vi "FG LED.vi"(2 "FG Action":T1, 3 "LED in":bool) -> (1 "LED out":bool)   [LabVIEW 2009]
uses:
  cRIO/Functional Global Variables/Actions for FG's.ctl
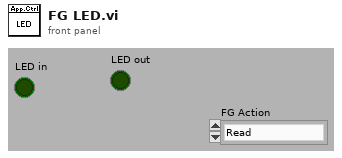
[diagram p1: front panel]
types:
  T1 = typedef "Actions for FG's.ctl" = enum16{"Read", "Write"}
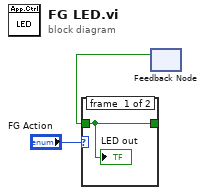
[diagram p0: block diagram]
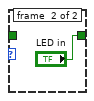
[diagram p2: hidden frame]
diagram:
  n1 = feedback #1() -> (w1:bool)  [unwired: 1 in]
  n2 = case shown="\"Read\", Default" "FG Action" {
    tunnel: [w4 "LED in"] -> w2
    tunnel: w1 -> [w4 _]
    frame #0 {
      "LED out" <- w4
    }
    frame #1 {
    }
  }
